vi "Begin.vi"(11 "Image Size":T1=enum."160x120") -> (0 "error out":errorcluster)   [LabVIEW 2012]
doc: "Called before other user functions, this VI is expected to open initial I/O refnums, load in file data, and do all program initialization. Notice that the <B>error out</B> terminal is simply used for data flow. Wiring it to other structures or subVIs ensures that this VI runs first."
uses:
  <vilib>/Rock Robotics/WPI/Camera/WPI_CameraImageSize.ctl
  <vilib>/Rock Robotics/WPI/Camera/WPI_CameraWhite Balance Values.ctl
  <vilib>/Rock Robotics/WPI/Camera/WPI_CameraExposure Values.ctl
  <vilib>/Rock Robotics/WPI/Camera/WPI_CameraFrameRate.ctl
  <vilib>/Rock Robotics/WPI/DriverStation/WPI_DriverStationRobotMode2.ctl
  <vilib>/Rock Robotics/SystemInterfaces/DIO/FPGA_DIOPWMChannel.ctl
  <vilib>/Rock Robotics/WPI/SafetyOutput/WPI_SafetyOutputConfigMenu.ctl
  <vilib>/Rock Robotics/WPI/Solenoid/WPI_SolenoidChannel.ctl
  <vilib>/Rock Robotics/SystemInterfaces/DIO/FPGA_DIOChannel.ctl
  <vilib>/Rock Robotics/SystemInterfaces/DIO/FPGA_DIORelayChannel.ctl
  <vilib>/Rock Robotics/WPI/Encoder/WPI_EncoderType.ctl
  <vilib>/Rock Robotics/WPI/Joystick/WPI_JoystickDeviceEnum.ctl
  Robot Global Data.vi
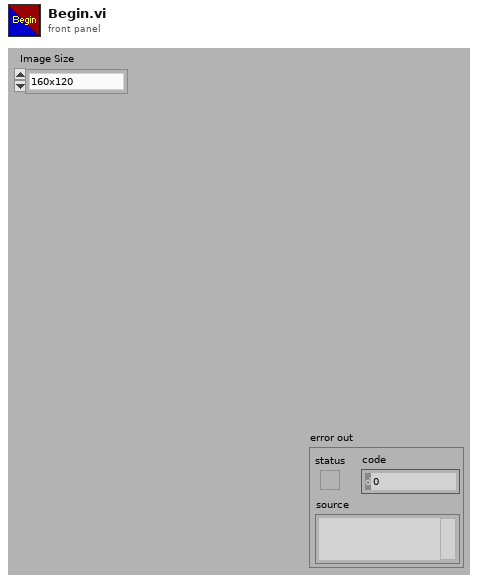
[diagram p1: front panel]
types:
  T1 = typedef "WPI_CameraImageSize.ctl" = enum16{"640x480", "320x240", "160x120"}
  T2 = typedef "FPGA_DIOChannel.ctl" = enum8{"DIO 1", "DIO 2", "DIO 3", "DIO 4", "DIO 5", "DIO 6", "DIO 7", "DIO 8", "DIO 9", "DIO 10", "DIO 11", "DIO 12", "DIO 13", "DIO 14", "Invalid"}
  T3 = typedef "WPI_SolenoidChannel.ctl" = enum8{"Solenoid 1", "Solenoid 2", "Solenoid 3", "Solenoid 4", "Solenoid 5", "Solenoid 6", "Solenoid 7", "Solenoid 8", "Invalid"}
  T4 = typedef "WPI_JoystickDeviceEnum.ctl" = enum16{"USB 1", "USB 2", "USB 3", "USB 4", "Kinect 1", "Kinect 2"}
  T5 = typedef "WPI_EncoderType.ctl" = enum16{"1x", "2x", "4x"}
  T6 = typedef "FPGA_DIORelayChannel.ctl" = enum8{"Relay 1", "Relay 2", "Relay 3", "Relay 4", "Relay 5", "Relay 6", "Relay 7", "Relay 8", "Invalid"}
  T7 = typedef "FPGA_DIOPWMChannel.ctl" = enum8{"PWM 1", "PWM 2", "PWM 3", "PWM 4", "PWM 5", "PWM 6", "PWM 7", "PWM 8", "PWM 9", "PWM 10", "Invalid"}
  T8 = typedef "WPI_SafetyOutputConfigMenu.ctl" = enum16{"Enable", "Disable"}
  T9 = typedef "WPI_DriverStationRobotMode2.ctl" = enum16{"Autonomous Disabled", "Autonomous Enabled", "Teleop Disabled", "Teleop Enabled", "Timeout", "Finish", "Test Disabled", "Test Enabled"}
  T10 = typedef "WPI_CameraFrameRate.ctl" = u32
  T11 = typedef "WPI_CameraExposure Values.ctl" = enum16{"Auto", "Flicker-free 50 Hz", "Flicker-free 60 Hz", "Hold current"}
  T12 = typedef "WPI_CameraWhite Balance Values.ctl" = enum16{"Auto", "Fixed indoor", "Fixed outdoor 1", "Fixed outdoor 2", "Fixed fluorescent 1", "Fixed fluorescent 2", "Hold current"}
  T13 = typedef "WPI_CameraDevRef.ctl" = cluster{"Camera Address":string, "CameraStatus":errorcluster, "Acquire Image Notifier":refnum<notifier>}
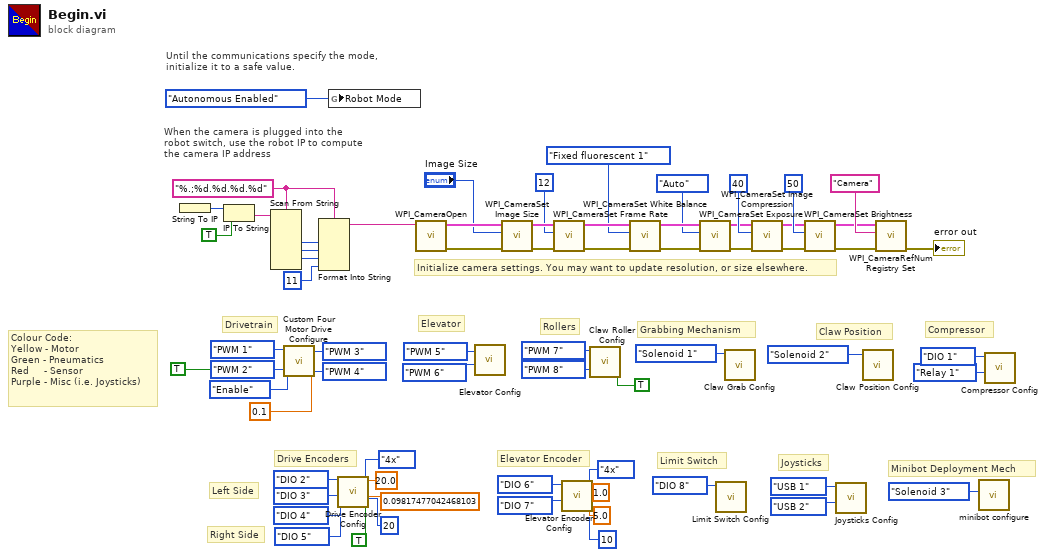
[diagram p0: block diagram]
diagram:
  w39 = "%.;%d.%d.%d.%d" ("format string")
  # "Limit Switch"
  # "Minibot Deployment Mech"
  # "Joysticks"
  # "Elevator Encoder"
  # "Compressor"
  # "Right Side"
  # "Left Side"
  # "Drive Encoders"
  # "Colour Code: \nYellow - Motor\nGreen - Pneumatics\nRed     - Sensor\nPurple - Misc (i.e. Joysticks)"
  # "Claw Position"
  # "Grabbing Mechanism"
  # "Rollers"
  # "Elevator"
  # "Drivetrain"
  # "Until the communications specify the mode,\ninitialize it to a safe value."
  # "When the camera is plugged into the\nrobot switch, use the robot IP to compute\nthe camera IP address"
  # "Initialize camera settings. You may want to update resolution, or size elsewhere."
  n1 = String To IP() -> (0:w46:u32)  [unwired: 1 in]
  n2 = IP To String(1:TRUE ("dot notation? (F)"), 2:w46) -> (0:w44:string)
  n3 = Scan From String(format string=w39, input string=w44) -> (output 1=w43:i32, output 2=w42:i32, output 3=w41:i32)  [unwired: 7 in, 3 out]
  n4 = call "Custom Four Motor Drive Configure.vi"("timeout (s)"=0.1, "Rear Right"=FPGA_DIOPWMChannel."PWM 4", "Front Right"=FPGA_DIOPWMChannel."PWM 3", "Safety Config State"=WPI_SafetyOutputConfigMenu."Enable", "Invert Right Side?"=TRUE, "Rear Left"=FPGA_DIOPWMChannel."PWM 2", "Front Left"=FPGA_DIOPWMChannel."PWM 1") -> ()  [unwired: 5 in]
  n5 = Format Into String(format string=w39, w43, w42, w41, 11 ("Compression")) -> (resulting string=w37:string)  [unwired: 2 in, 1 out]
  n6 = global write "Robot Global Data.vi" "Robot Mode"(WPI_DriverStationRobotMode2."Autonomous Enabled" ("Robot Mode")) -> ()
  n7 = call "Drive Encoder Config.vi"("Left Drive Encoder Channel A"=FPGA_DIOChannel."DIO 2", "Decoding Type"=WPI_EncoderType."4x", "Left Drive Encoder Channel B"=FPGA_DIOChannel."DIO 3", "Minimum Rate"=20.0, "DistancePerCount"=0.09817477042468103, "Right Drive Encoder Channel A"=FPGA_DIOChannel."DIO 4", "Number Samples to Average"=u8 20, "Right Drive Encoder Channel B"=FPGA_DIOChannel."DIO 5", "Invert Right Side"=TRUE) -> ()  [unwired: 7 in]
  n8 = call <vilib>:"WPI_CameraOpen.vi"("Camera Address"=w37) -> ("error out"=w58:errorcluster, "CameraDevRef"=w59:T13)  [unwired: 1 in, 8 out]
  n9 = call "Elevator Config.vi"("Elevator Bottom"=FPGA_DIOPWMChannel."PWM 6" ("Elevator Right"), "Elevator Top"=FPGA_DIOPWMChannel."PWM 5" ("Elevator Left")) -> ()  [unwired: 10 in]
  n10 = call <vilib>:"WPI_CameraSet Image Size.vi"("error in (no error)"=w58, "Image Size"="Image Size", "CameraDevRef"=w59) -> ("error out"=w57:errorcluster, "CameraDevRef Out"=w60:T13)  [unwired: 7 out]
  n11 = call <vilib>:"WPI_CameraSet Frame Rate.vi"("error in (no error)"=w57, "Frame Rate (fps)"=T10 12, "CameraDevRef"=w60) -> ("error out"=w56:errorcluster, "CameraDevRef Out"=w62:T13)  [unwired: 7 out]
  n12 = call "Elevator Encoder Config.vi"("Number Samples to Average"=u8 10, "Minimum Rate"=5.0, "DistancePerCount"=1.0, "Decoding Type"=WPI_EncoderType."4x", "Channel B"=FPGA_DIOChannel."DIO 7", "Channel A"=FPGA_DIOChannel."DIO 6") -> ()  [unwired: 6 in]
  n13 = call "Claw Roller Config.vi"("Invert"=TRUE, "Roller Right"=FPGA_DIOPWMChannel."PWM 8", "Roller Left"=FPGA_DIOPWMChannel."PWM 7") -> ()  [unwired: 9 in]
  n14 = call <vilib>:"WPI_CameraSet White Balance.vi"("error in (no error)"=w56, "White Balance"=WPI_CameraWhite_Balance_Values."Fixed fluorescent 1", "CameraDevRef"=w62) -> ("error out"=w55:errorcluster, "CameraDevRef Out"=w61:T13)  [unwired: 7 out]
  n15 = call <vilib>:"WPI_CameraSet Exposure.vi"("error in (no error)"=w55, "Exposure"=WPI_CameraExposure_Values."Auto", "CameraDevRef"=w61) -> ("error out"=w54:errorcluster, "CameraDevRef Out"=w64:T13)  [unwired: 7 out]
  n16 = call "Limit Switch Config.vi"("DIO Channel"=FPGA_DIOChannel."DIO 8") -> ()  [unwired: 11 in]
  n17 = call "Claw Grab Config.vi"("Solenoid Channel"=WPI_SolenoidChannel."Solenoid 1") -> ()  [unwired: 11 in]
  n18 = call <vilib>:"WPI_CameraSet Image Compression.vi"("error in (no error)"=w54, "Compression"=40, "CameraDevRef"=w64) -> ("error out"=w53:errorcluster, "CameraDevRef Out"=w63:T13)  [unwired: 7 out]
  n19 = call <vilib>:"WPI_CameraSet Brightness.vi"("error in (no error)"=w53, "Brightness"=50, "CameraDevRef"=w63) -> ("error out"=w51:errorcluster, "CameraDevRef Out"=w52:T13)  [unwired: 7 out]
  n20 = call "Joysticks Config.vi"("Secondary Controller USB Output"=WPI_JoystickDeviceEnum."USB 2", "Primary Controller Usb Output"=WPI_JoystickDeviceEnum."USB 1") -> ()  [unwired: 10 in]
  n21 = call "Claw Position Config.vi"("Claw Position"=WPI_SolenoidChannel."Solenoid 2") -> ()  [unwired: 11 in]
  n22 = call <vilib>:"WPI_CameraRefNum Registry Set.vi"("error in (no error)"=w51, "refnum name"="Camera", "CameraDevRef"=w52) -> ("error out"=→"error out":errorcluster)  [unwired: 8 out]
  n23 = call "minibot configure.vi"("Solenoid Channel"=WPI_SolenoidChannel."Solenoid 3") -> ()  [unwired: 11 in]
  n24 = call "Compressor Config.vi"("Relay Channel"=FPGA_DIORelayChannel."Relay 1", "Pressure Switch DIO Channel"=FPGA_DIOChannel."DIO 1") -> ()  [unwired: 10 in]
